vi "Increment Bytes Received.vi"(8 "error in (no error)":errorcluster, 10 "Increment":i32, 11 "TCP_Server_Connection_Handler in":refnum<class "TCP_Server_Connection_Handler.lvclass">) -> (0 "error out":errorcluster, 3 "TCP_Server_Connection_Handler out":refnum<class "TCP_Server_Connection_Handler.lvclass">)   [LabVIEW 2023, in "TCP_Server_Connection_Handler.lvlib" / "TCP_Server_Connection_Handler.lvclass"]
uses:
  TCP_Server_Connection_Handler.lvclass
  <vilib>/ActorFramework/Actor/Actor.lvclass
  TCP_Connections_Controller Messages/ConnectionInfoUpdated Msg/ConnectionInfoUpdated Msg.lvclass
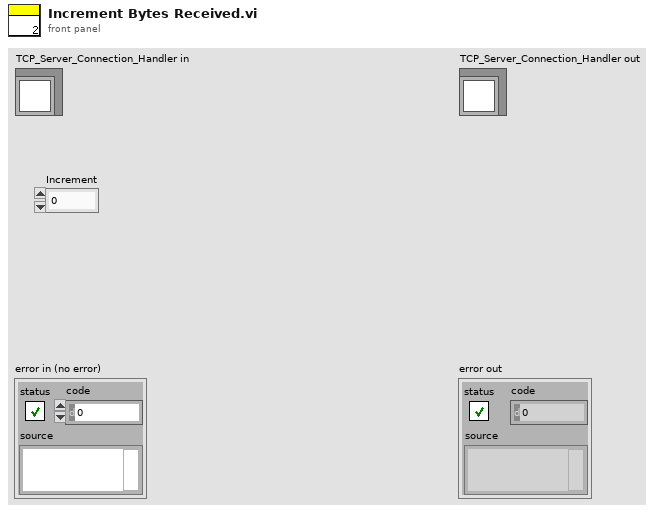
[diagram p1: front panel]
types:
  T1 = typedef "TCP_Listener.lvlib/ConnectionInformation.ctl" = cluster{"Connection number":i32, "Remote Address":string, "Remote Port":u16, "Connection ID":refnum<k5>, "bytes received":i32, "bytes  sent":i32}
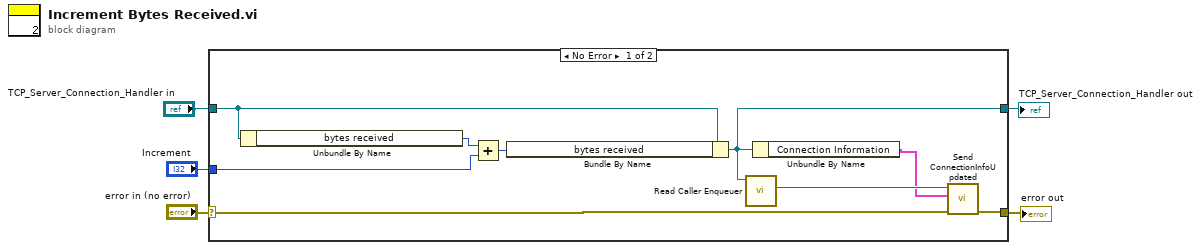
[diagram p0: block diagram]
diagram:
  n1 = case shown="No Error" "error in (no error)" {
    selector: "error in (no error)" -> [w7 w16]
    tunnel: [w6 w16] -> w4
    tunnel: [w10 w15] -> w2
    tunnel: "TCP_Server_Connection_Handler in" -> [w12 w15]
    tunnel: "Increment" -> [w13 _]
    frame No Error {
      n2 = Unbundle By Name(w12) -> ("bytes received"=w14:i32)
      n3 = Add(x=w14, y=w13) -> (x+y=w11:i32)
      n4 = Bundle By Name(cluster=w12, "bytes received"=w11) -> (w10:refnum<class "TCP_Server_Connection_Handler.lvclass">)
      n5 = call <vilib>:"Read Caller Enqueuer.vi"("Actor"=w10) -> ("Caller Enqueuer"=w9:refnum<class "Message Enqueuer.lvclass">)  [unwired: 10 in]
      n6 = Unbundle By Name(w10) -> ("Connection Information"=w8:T1)
      n7 = call "Send ConnectionInfoUpdated.vi"("error in (no error)"=w7, "Connection Information"=w8, "Message Enqueuer"=w9) -> ("error out"=w6:errorcluster)  [unwired: 7 in, 1 out]
    }
    frame Error {
    }
  }
  "error out" <- w4
  "TCP_Server_Connection_Handler out" <- w2
